vi "Write State Machine State.vi"(8 "error in (no error)":errorcluster, 10 "Command Processor State":T1, 11 "Command Processor Actor in":refnum<class "Command Processor Actor.lvclass">) -> (0 "error out":errorcluster, 3 "Command Processor Actor out":refnum<class "Command Processor Actor.lvclass">)   [LabVIEW 2014, in "Robot Actor Framework.lvlib" / "Command Processor Actor.lvlib" / "Command Processor Actor.lvclass"]
uses:
  Command Processor Actor.lvclass
  Command Processor States.ctl
  Command Processor Actor.lvclass/Command Processor Actor.ctl
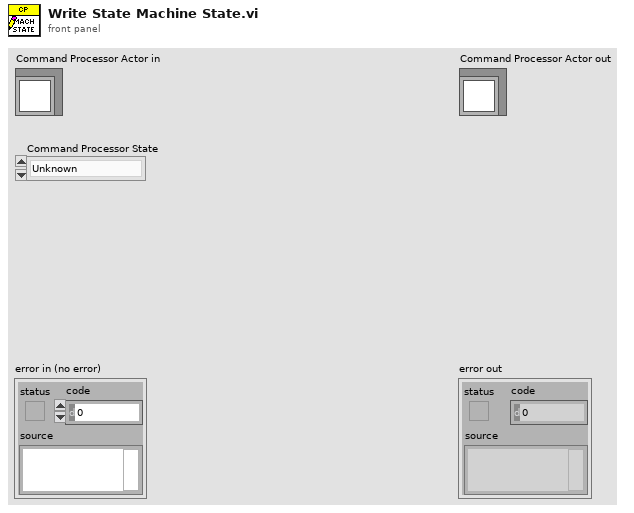
[diagram p1: front panel]
types:
  T1 = typedef "Robot Actor Framework.lvlib/Command Processor Actor.lvlib/Command Processor Actor.lvclass/Command Processor States.ctl" = enum16{"Unknown", "No Command", "Running Command", "Starting Command", "Stopping Command", "Finishing Command"}
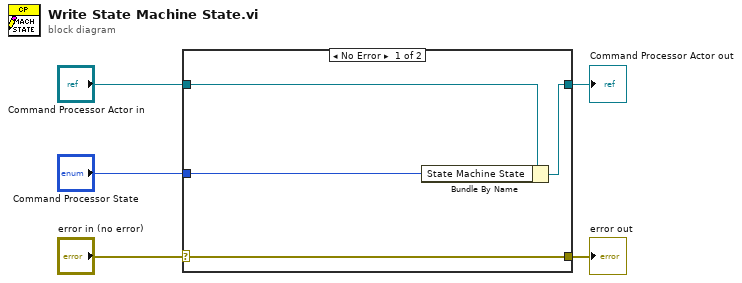
[diagram p0: block diagram]
diagram:
  n1 = case shown="No Error" "error in (no error)" {
    selector: "error in (no error)" -> [w9 w10]
    tunnel: [w9 w10] -> w4
    tunnel: [w7 w11] -> w2
    tunnel: "Command Processor Actor in" -> [w8 w11]
    tunnel: "Command Processor State" -> [w6 _]
    frame No Error {
      n2 = Bundle By Name(cluster=w8, "State Machine State"=w6) -> (w7:refnum<class "Command Processor Actor.lvclass">)
    }
    frame Error {
    }
  }
  "error out" <- w4
  "Command Processor Actor out" <- w2
